vi "Stop.vi"(8 "error in (no error)":errorcluster, 11 "CodeCoverage in":refnum<class "CodeCoverage.lvclass">) -> (0 "error out":errorcluster, 3 "CodeCoverage out":refnum<class "CodeCoverage.lvclass">)   [LabVIEW 2017, in "CodeCoverage.lvclass"]
doc: "Stops code coverage measurement and clears the context."
uses:
  CodeCoverage.lvclass
  CodeCoverage.lvclass/CodeCoverage.ctl
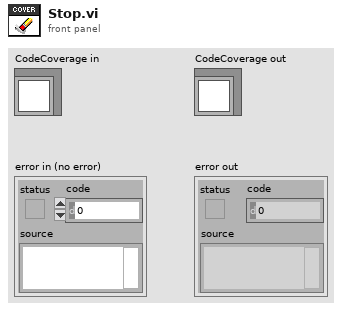
[diagram p1: front panel]
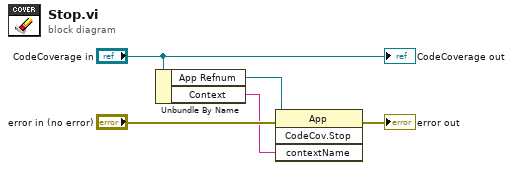
[diagram p0: block diagram]
diagram:
  n1 = Unbundle By Name("CodeCoverage in") -> ("App Refnum"=w3:refnum<vi>, "Context"=w1:string)
  n2 = invoke class="App" method="CodeCov.Stop"(reference=w3, error in="error in (no error)", "contextName"=w1) -> (error out=→"error out":errorcluster)  [unwired: 1 in, 3 out]
  "CodeCoverage out" <- "CodeCoverage in"
